vi "Move Data to new file.vi"() -> ()   [LabVIEW 2015]
panel:
  in  "channel name(s) in":string[](array[string])
  in  "Dest File":path
  in  "Starting file":path
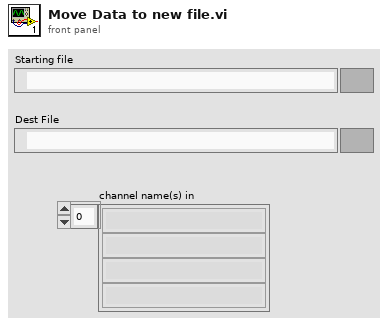
[diagram p1: front panel]
types:
  T1 = enum16{"open", "open or create", "create or replace", "create", "open (read-only)"}
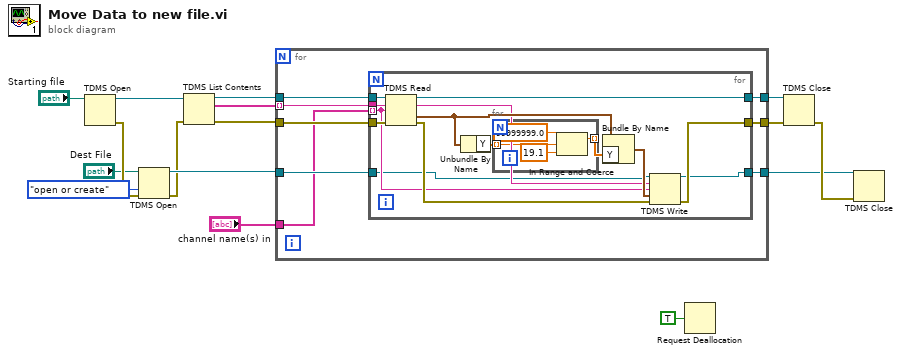
[diagram p0: block diagram]
diagram:
  n1 = TDMS Open(11:"Starting file") -> (0:w16:errorcluster, 3:w7:refnum<k34>)  [unwired: 6 in]
  n2 = TDMS Open(8:w16, 10:T1."open or create" ("operation (0:open)"), 11:"Dest File") -> (0:w6:errorcluster, 3:w12:refnum<k34>)  [unwired: 4 in]
  n3 = TDMS List Contents(4:w6, 7:w7) -> (0:w5:errorcluster, 2:w3:string[], 3:w4:refnum<k34>)  [unwired: 1 in, 1 out]
  n4 = for {
    tunnel: w3 -> [w18] mode=indexing
    tunnel: w4 -> [w19]
    tunnel: [w23] -> w13
    tunnel: w12 -> [w22]
    tunnel: [w21] -> w11
    tunnel: w5 -> [w20]
    tunnel: [w24] -> w15
    tunnel: "channel name(s) in" -> [w17]
    n5 = for {
      tunnel: w18 -> [w28]
      tunnel: w19 -> [w35]
      tunnel: [w37] -> w23
      tunnel: w22 -> [w26]
      tunnel: [w25] -> w21
      tunnel: w20 -> [w36]
      tunnel: [w30] -> w24
      tunnel: w17 -> [w27] mode=indexing
      n6 = TDMS Read(0:w35, 5:w28, 7:w27, 11:w36) -> (4:w37:refnum<k34>, 10:w33:waveform(dbl), 15:w31:errorcluster)  [unwired: 4 in, 3 out]
      n7 = Unbundle By Name(w33) -> ("Y"=w34:dbl[])
      n8 = for {
        tunnel: w34 -> [w41] mode=indexing
        tunnel: [w38] -> w32 mode=indexing
        n9 = In Range and Coerce(upper limit=99999999.0, x=w41, lower limit=19.1) -> (coerced(x)=w38:dbl)  [unwired: 1 out]
      }
      n10 = Bundle By Name(cluster=w33, "Y"=w32) -> (w29:waveform(dbl))
      n11 = TDMS Write(0:w26, 5:w28, 7:w27, 9:w29, 11:w31) -> (4:w25:refnum<k34>, 15:w30:errorcluster)  [unwired: 1 in, 2 out]
    }
  }
  n12 = Request Deallocation(TRUE ("flag")) -> ()
  n13 = TDMS Close(8:w15, 11:w13) -> (0:w14:errorcluster)  [unwired: 1 out]
  n14 = TDMS Close(8:w14, 11:w11) -> ()  [unwired: 2 out]
